vi "Compute Offset.vi"(11 "C&C Data in":T1={"Hardware Configuration"={"COM Port"="", "Reference Distance"=0.0, "Sensor SN"=""}, "Logging Configuration"={"Log File Base Path"=path "", "Datafile Ref"=refnum, "Database Ref"=refnum}, "UI Refs"={"Start Ref"=refnum, "Settings Ref"=refnum, "Stop Ref"=refnum, "Exit Ref"=refnum, "Status Ref"=refnum, "Data Ref"=refnum, "StatusBox Ref"=refnum, "Location Ref"=refnum, "Operator Ref"=refnum, "Time Ref"=refnum, "Test in Progess Ref"=refnum}, "Calibration Data"={"calibrationID"=0, "operatorID"=0, "sensorID"=0, "start_time"="", "end_time"="", "offset"=0.0, "offset_units"="", "ring_time"=0.0, "error"=0.0, "Passed"=0, "data_storage_location"="", "comments"=""}, "Time Elapsed"=0, "Samples Required"=480} {"Hardware Configuration"."Reference Distance" format="%.3g"}) -> (1 "Test Results":string, 2 "Test Result Array":string[](array[string]), 3 "C&C Data out":T1={"Hardware Configuration"={"COM Port"="", "Reference Distance"=0.0, "Sensor SN"=""}, "Logging Configuration"={"Log File Base Path"=path "", "Datafile Ref"=refnum, "Database Ref"=refnum}, "UI Refs"={"Start Ref"=refnum, "Settings Ref"=refnum, "Stop Ref"=refnum, "Exit Ref"=refnum, "Status Ref"=refnum, "Data Ref"=refnum, "StatusBox Ref"=refnum, "Location Ref"=refnum, "Operator Ref"=refnum, "Time Ref"=refnum, "Test in Progess Ref"=refnum}, "Calibration Data"={"calibrationID"=0, "operatorID"=0, "sensorID"=0, "start_time"="", "end_time"="", "offset"=0.0, "offset_units"="", "ring_time"=0.0, "error"=0.0, "Passed"=0, "data_storage_location"="", "comments"=""}, "Time Elapsed"=0, "Samples Required"=480} {"Hardware Configuration"."Reference Distance" format="%.3g"})   [LabVIEW 2018]
uses:
  Settings/Settings.ctl
  Acquisition/Hardware Configuration.ctl
  Logging/Logging Configuration.ctl
  <vilib>/addons/database/Connection.llb/Conn ObjectReference.ctl
  Controls/Location Ring.ctl
  Controls/Time Remaining.ctl
  Acquisition/Acquisition.lvlib
  <vilib>/addons/database/NI_Database_API.lvlib
  Logging/Logging.lvlib
  Settings/Settings.lvlib
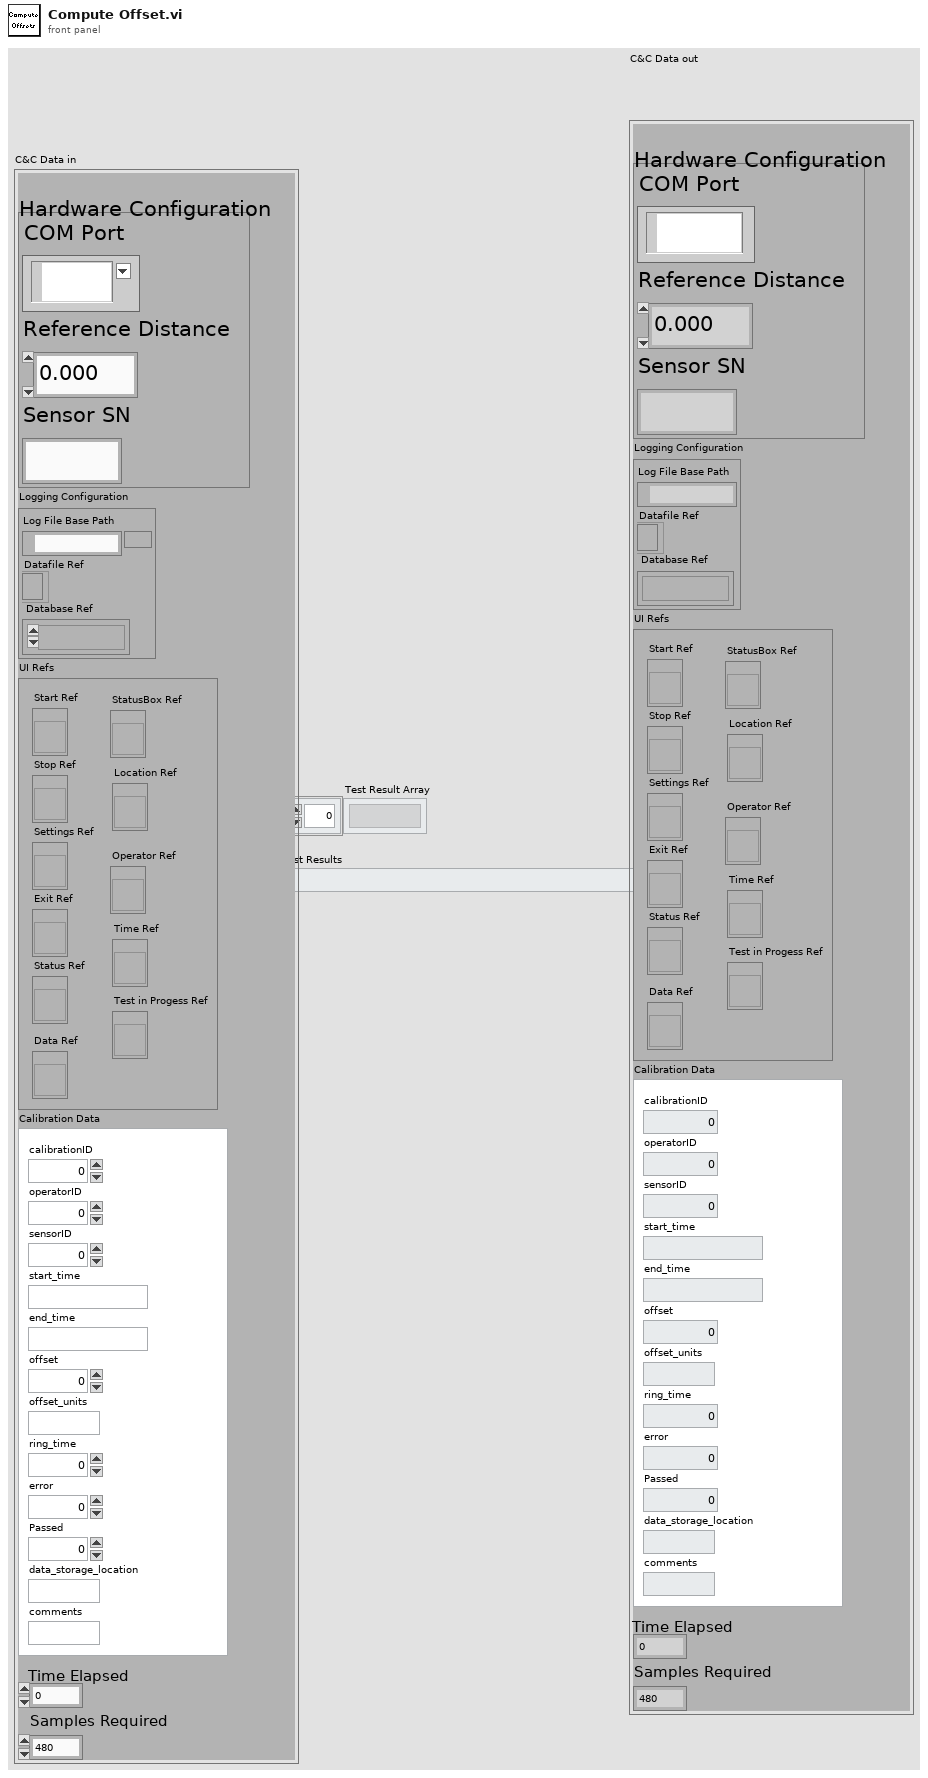
[diagram p1: front panel]
types:
  T1 = typedef "Settings.lvlib/Settings.ctl" = cluster{"Hardware Configuration":T2, "Logging Configuration":T3, "UI Refs":cluster{"Start Ref":refnum<vi>, "Settings Ref":refnum<vi>, "Stop Ref":refnum<vi>, "Exit Ref":refnum<vi>, "Status Ref":refnum<vi>, "Data Ref":refnum<vi>, "StatusBox Ref":refnum<vi>, "Location Ref":refnum<vi>, "Operator Ref":refnum<vi>, "Time Ref":refnum<vi>, "Test in Progess Ref":refnum<vi>}, "Calibration Data":cluster{"calibrationID":u16, "operatorID":u16, "sensorID":u16, "start_time":string, "end_time":string, "offset":dbl, "offset_units":string, "ring_time":dbl, "error":dbl, "Passed":u8, "data_storage_location":string, "comments":string}, "Time Elapsed":u16, "Samples Required":u16}
  T2 = typedef "Acquisition.lvlib/Hardware Configuration.ctl" = cluster{"COM Port":refnum<visa-resource-name>, "Reference Distance":dbl, "Sensor SN":string}
  T3 = typedef "Logging.lvlib/Logging Configuration.ctl" = cluster{"Log File Base Path":path, "Datafile Ref":refnum<file>, "Database Ref":T4}
  T4 = typedef "NI_Database_API.lvlib/Conn ObjectReference.ctl" = refnum<k1>
  T5 = cluster{"calibrationID":u16, "operatorID":u16, "sensorID":u16, "start_time":string, "end_time":string, "offset":dbl, "offset_units":string, "ring_time":dbl, "error":dbl, "Passed":u8, "data_storage_location":string, "comments":string}
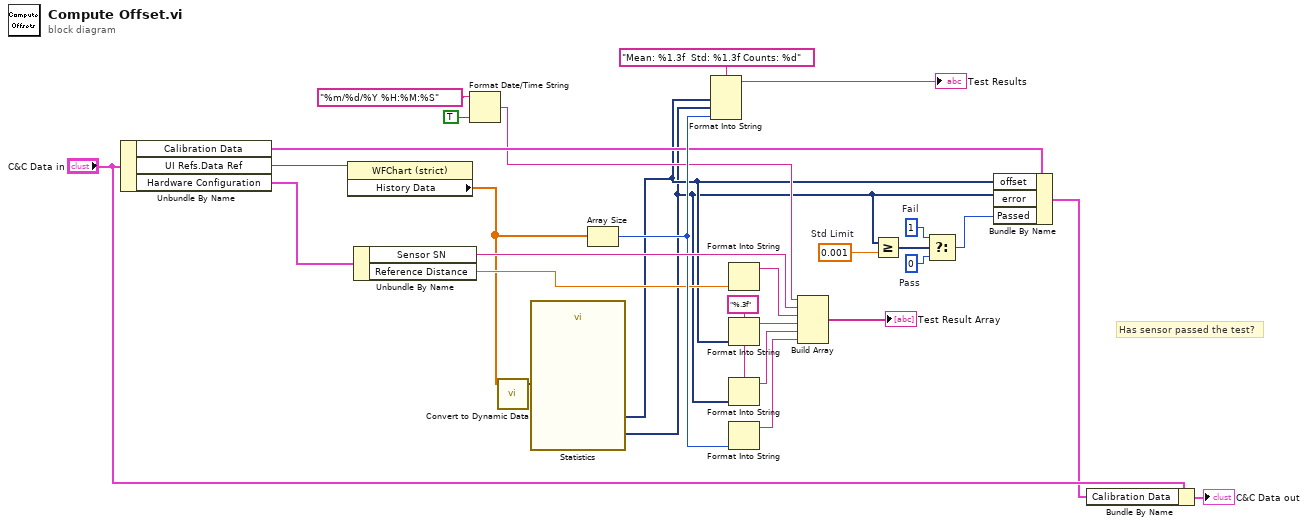
[diagram p0: block diagram]
diagram:
  w8 = 0.001  # Std Limit
  w11 = u8 1  # Fail
  w12 = u8 0  # Pass
  w23 = "%.3f" ("format string")
  # "Has sensor passed the test?"
  n1 = Unbundle By Name("C&C Data in") -> ("Calibration Data"=w16:T5, "UI Refs.Data Ref"=w18:refnum<vi>, "Hardware Configuration"=w17:T2)
  n2 = property on="Data Values" class="WFChart (strict)"(reference=w18) -> ("History Data"=w4:dbl[])  [unwired: 1 in, 2 out]
  n3 = Unbundle By Name(w17) -> ("Sensor SN"=w24:string, "Reference Distance"=w21:dbl)
  n4 = Format Date/Time String(time format string (%c)="%m/%d/%Y %H:%M:%S" ("string"), UTC format=TRUE) -> (date/time string=w5:string)  [unwired: 1 in]
  n5 = call "Convert to Dynamic Data"("Array"=w4) -> ("Dynamic Data Type"=w3:dynamicdata)  [unwired: 3 in]
  n6 = call "Statistics"("Signals"=w3) -> ("Standard Dev"=w1:dynamicdata, "Arithmetic Mean"=w2:dynamicdata)  [unwired: 24 in, 1 out]
  n7 = Array Size(array=w4) -> (size(s)=w22:i32)
  n8 = Format Into String(format string="Mean: %1.3f  Std: %1.3f Counts: %d", w2, w1, w22) -> (resulting string=→"Test Results":string)  [unwired: 2 in, 1 out]
  n9 = Format Into String(w21) -> (resulting string=w25:string)  [unwired: 3 in, 1 out]
  n10 = Format Into String(format string=w23, w2) -> (resulting string=w26:string)  [unwired: 2 in, 1 out]
  n11 = Format Into String(format string=w23, w1) -> (resulting string=w27:string)  [unwired: 2 in, 1 out]
  n12 = Format Into String(w22) -> (resulting string=w28:string)  [unwired: 3 in, 1 out]
  n13 = Build Array(w5, w24, w25, w26, w27, w28) -> (→"Test Result Array":string[])
  n14 = Greater Or Equal?(x=w1, y=w8) -> (x >= y?=w9:dynamicdata)
  n15 = Select(t=w11, s=w9, f=w12) -> (s? t:f=w10:u8)
  n16 = Bundle By Name(cluster=w16, "offset"=w2, "error"=w1, "Passed"=w10) -> (w14:T5)
  n17 = Bundle By Name(cluster="C&C Data in", "Calibration Data"=w14) -> (→"C&C Data out":T1)
